vi "UI Allmotion.vi"(8 "error in":errorcluster) -> (0 "error out":errorcluster)   [LabVIEW 2019, in "Allmotion.lvlib"]
uses:
  Allmotion.lvlib
  User Event/Controls/UE Abort Action.ctl
  <vilib>/Utility/miscctls.llb/LVPointTypeDef.ctl
  <vilib>/Utility/error.llb/Error Cluster From Error Code.vi
  <vilib>/Instr/_visa.llb/VISA Configure Serial Port (Instr).vi
  <vilib>/Utility/config.llb/Read Key (String).vi
  <vilib>/ErrorRing/Error Ring.xnode
  Queues/Queues.lvlib
  <vilib>/Utility/config.llb/NI_LVConfig.lvlib
panel:
  in  "Cube":T1(radio)=enum."Cube 1"
  in  "Go Reference":bool
  in  "Joystick Control":T2={"Joystick"=FALSE, "Deadband"={"Axis 1"=2000, "Axis 2"=2000, "Axis 3"=500}, "Multiply"={"Axis 1"=100, "Axis 2"=100, "Axis 3"=25}}
  in  "EMC":bool
  in  "Reset":bool
  in  "Home":bool
  in  "Motion Control":T3
  out "Current Position":i32[](array[numeric])
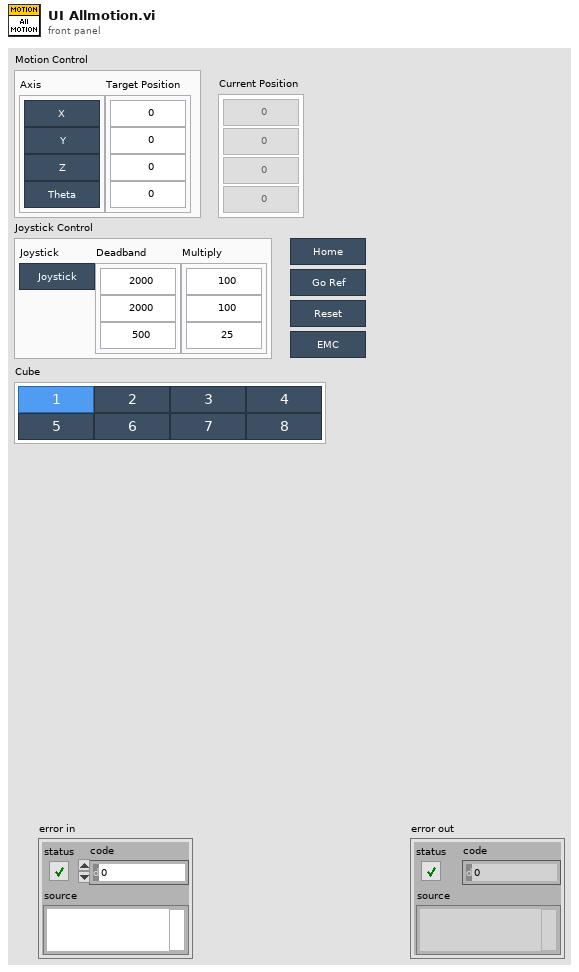
[diagram p1: front panel]
types:
  T1 = enum32{"No Selection", "Cube 1", "Cube 2", "Cube 3", "Cube 4", "Cube 5", "Cube 6", "Cube 7", "Cube 8"}
  T2 = cluster{"Joystick":bool, "Deadband":cluster{"Axis 1":i32, "Axis 2":i32, "Axis 3":i32}, "Multiply":cluster{"Axis 1":i32, "Axis 2":i32, "Axis 3":i32}}
  T3 = cluster{"Axis":cluster{"X":bool, "Y":bool, "Z":bool, "Theta":bool}, "Target Position":cluster{"X":i32, "Y":i32, "Z":i32, "Theta":i32}}
  T4 = cluster{"VISA name":refnum<visa-resource-name>, "Dichroic Position":string[], "Reference":string[]}
  T5 = typedef "UE Abort Action.ctl" = enum16{"Create", "Get", "Destroy"}
  T6 = typedef "LVPointTypeDef.ctl" = cluster{"Horizontal":i16, "Vertical":i16}
  T7 = enum8{"Enabled", "Disabled", "Disabled and Grayed Out"}
  T8 = typedef "NI_LVConfig.lvlib/Config Data RefNum.ctl" = refnum<k1>
  T9 = typedef "Allmotion.lvlib/SEQ Data.ctl" = cluster{"Position":i32[], "Arrived?":bool, "VISA name":refnum<visa-resource-name>, "Initialize Done?":bool, "State":string, "VI Refnum":refnum<vi>, "Dichroic Position":string[]}
  T10 = typedef "Rendezvous RefNum" = refnum<k1>
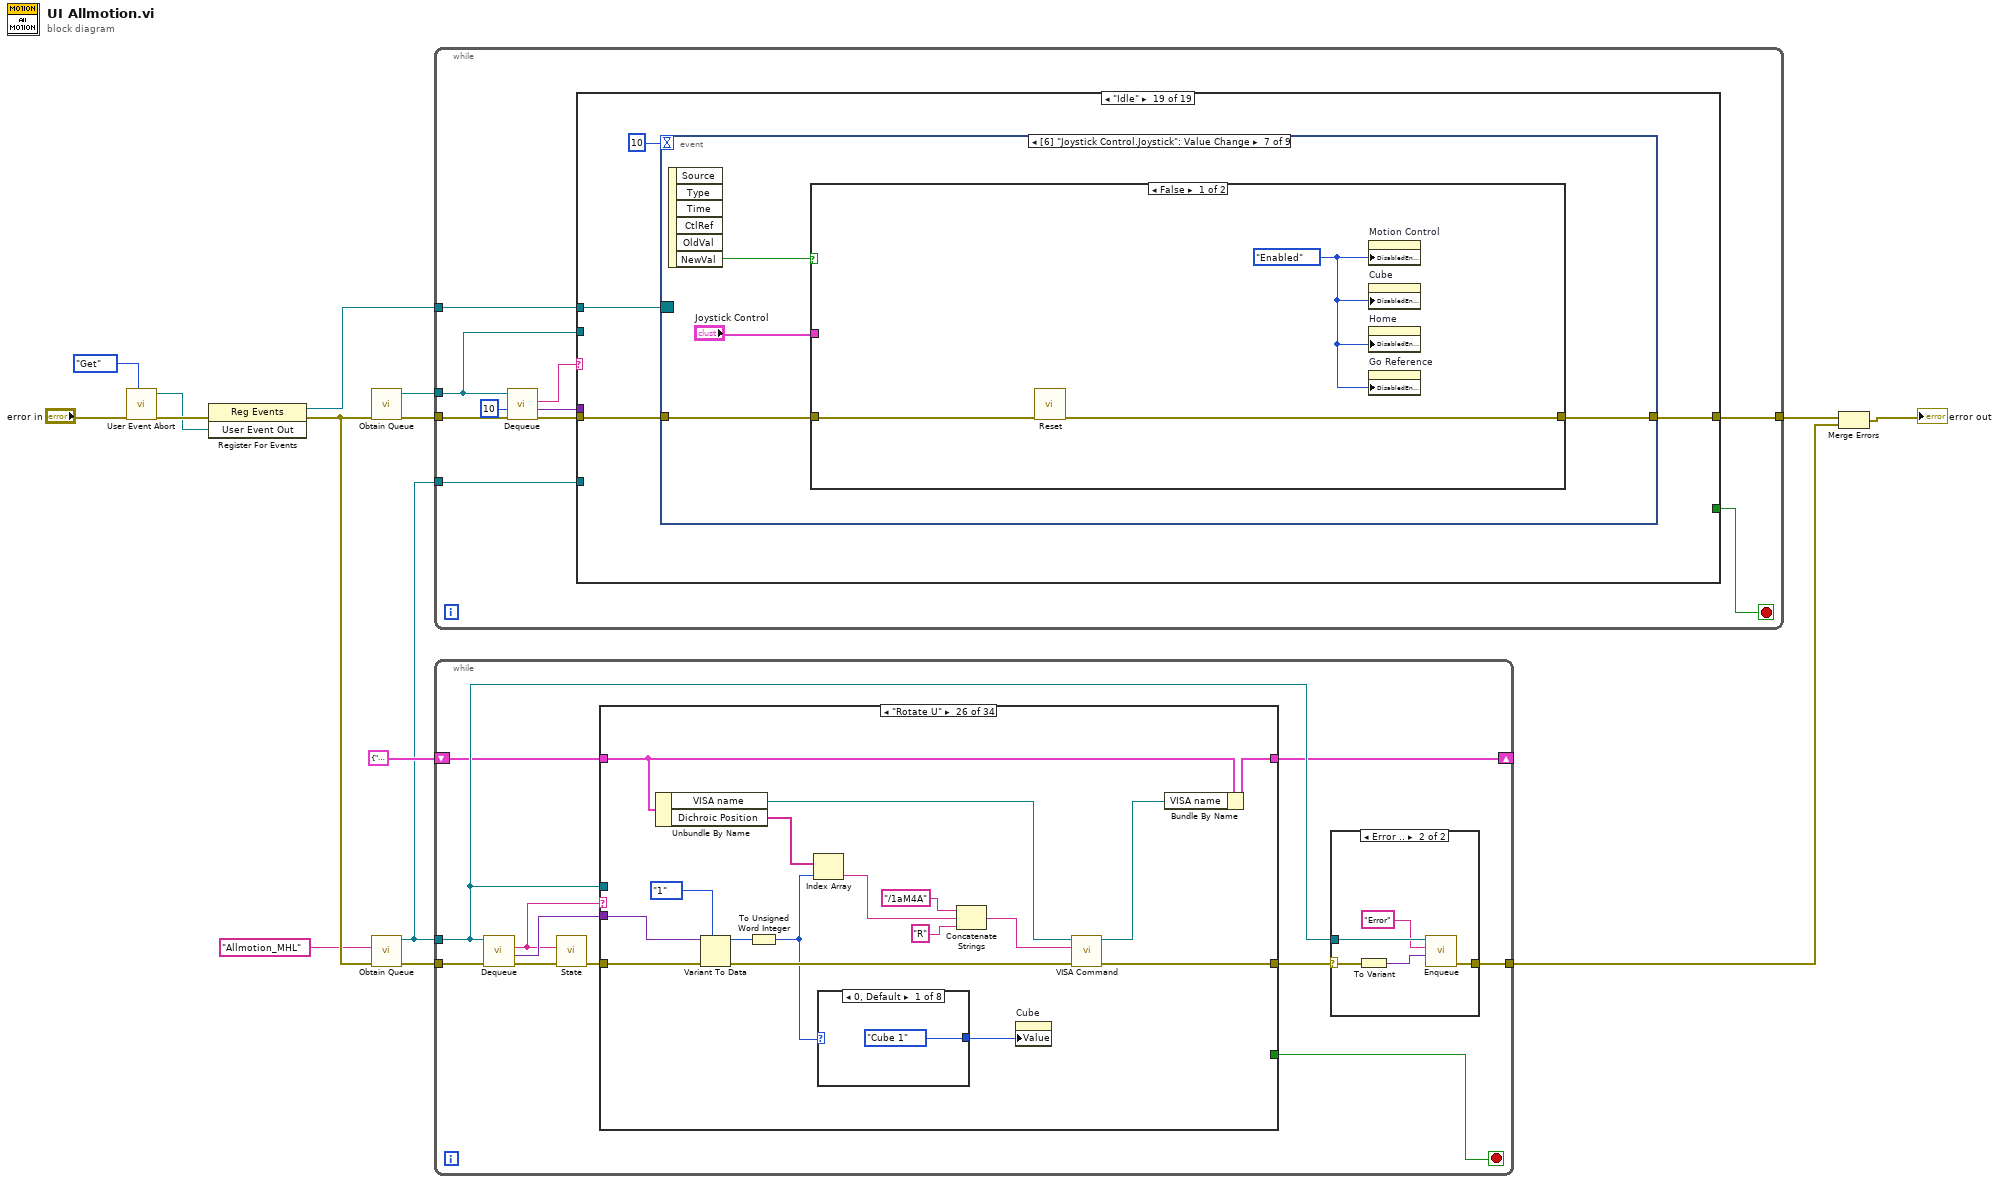
[diagram p0: block diagram]
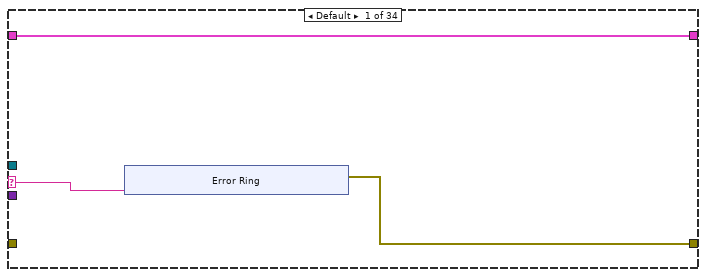
[diagram p3: hidden frame]
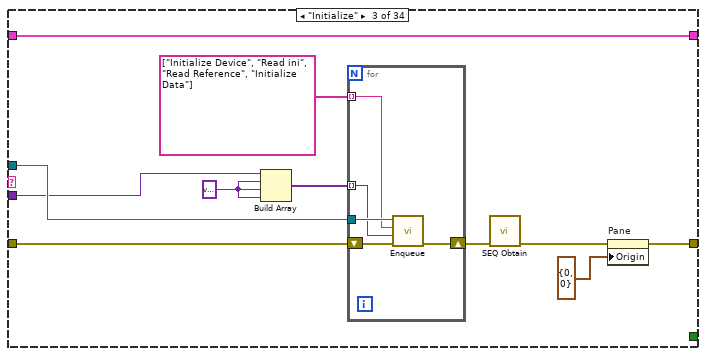
[diagram p5: hidden frame]
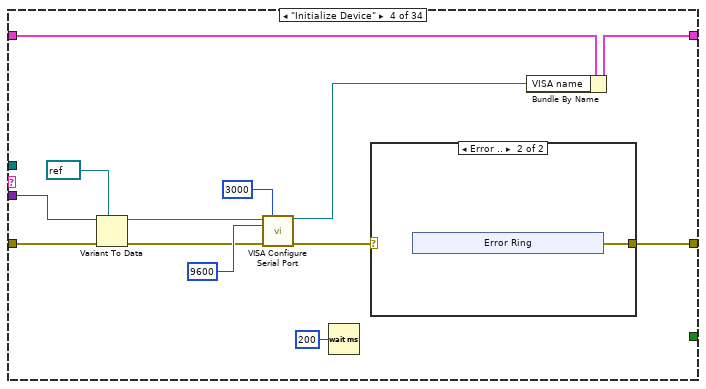
[diagram p6: hidden frame]
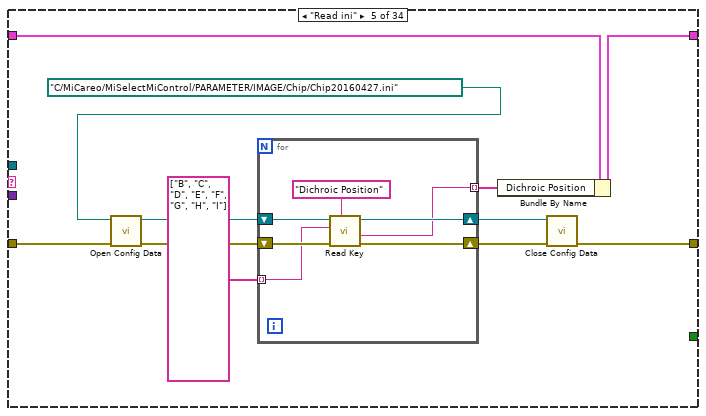
[diagram p8: hidden frame]
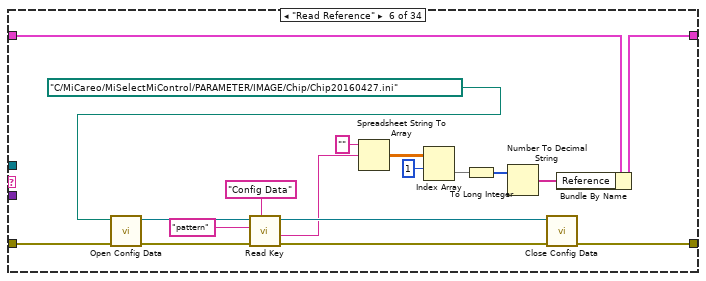
[diagram p9: hidden frame]
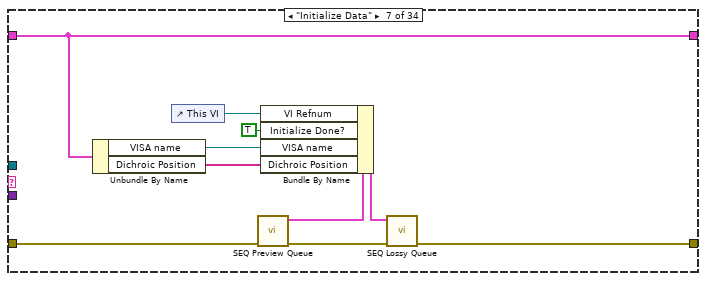
[diagram p10: hidden frame]
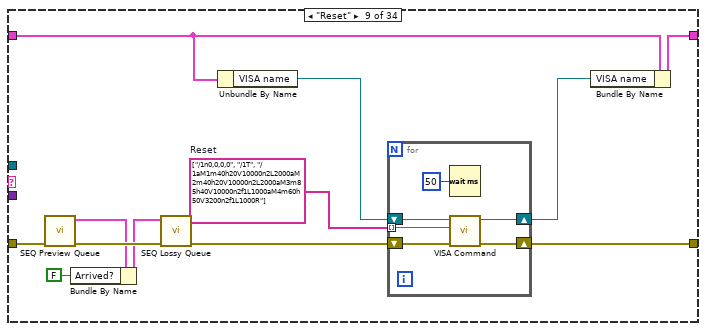
[diagram p12: hidden frame]
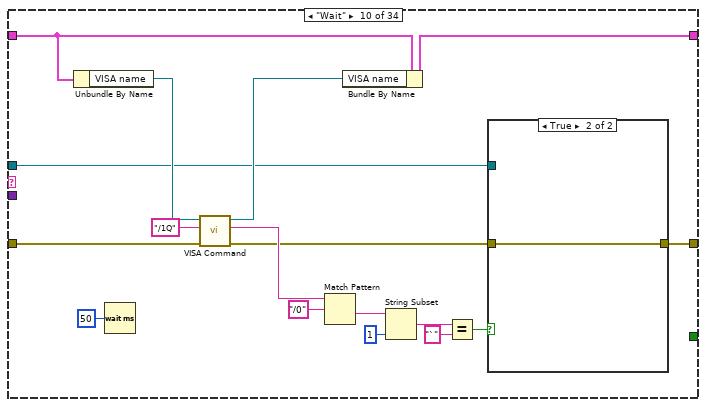
[diagram p13: hidden frame]
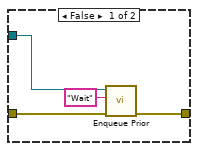
[diagram p14: hidden frame]
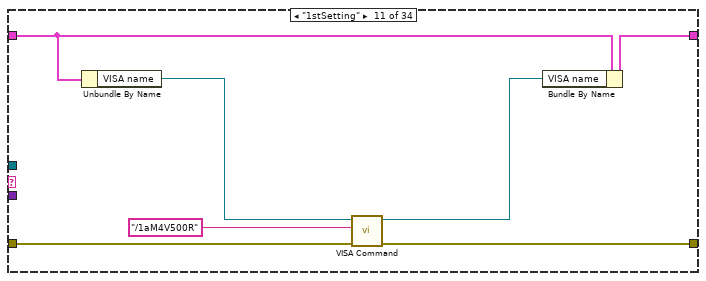
[diagram p15: hidden frame]
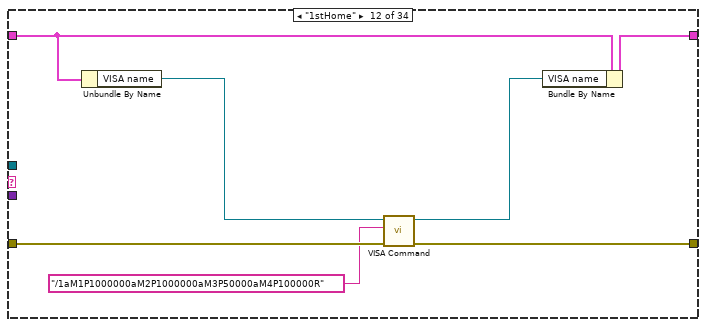
[diagram p16: hidden frame]
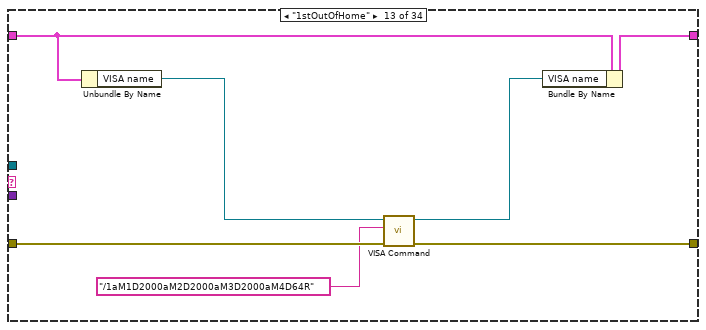
[diagram p17: hidden frame]
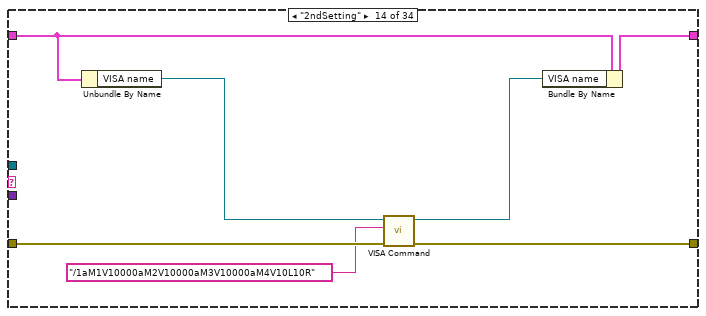
[diagram p18: hidden frame]
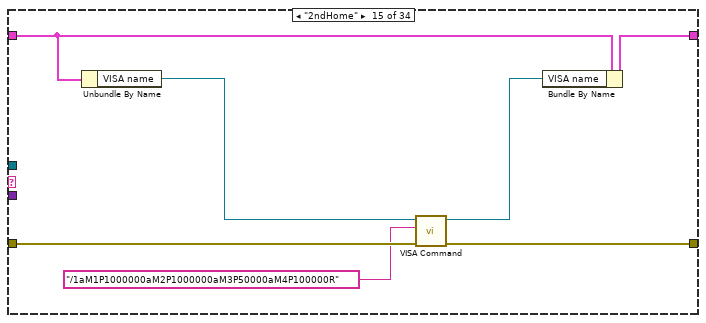
[diagram p19: hidden frame]
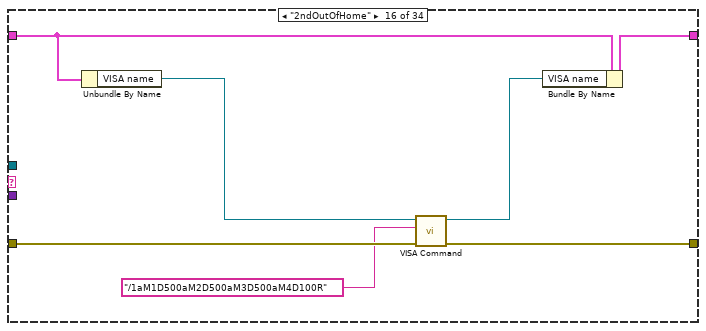
[diagram p20: hidden frame]
diagram:
  n1 = call "User Event Abort.vi"("Action"=UE_Abort_Action."Get", "Error In"="error in") -> ("Error Out"=w13:errorcluster, "User Event Out"=w12:refnum<user-event>)  [unwired: 8 in]
  n2 = register-events(error in=w13, w12) -> (reference out=w11:refnum<event-registration>, error out=w4:errorcluster)  [unwired: 1 in]
  n3 = call "Obtain Queue.vi"("Error In"=w4) -> ("Error Out"=w6:errorcluster, "Queue out"=w5:refnum<queue>)  [unwired: 9 in]
  n4 = call "Obtain Queue.vi"("Error In"=w4, "Queue Name"="Allmotion_MHL") -> ("Error Out"=w3:errorcluster, "queue out"=w2:refnum<queue>)  [unwired: 8 in]
  n5 = while {
    tunnel: w6 -> [w25]
    tunnel: w11 -> [w20]
    tunnel: [w19] -> w10
    tunnel: w2 -> [w17]
    tunnel: w5 -> [w16]
    stop <- w18 stop-if-true
    n6 = call "Dequeue.vi"("Error In"=w25, "timeout in ms (-1)"=10, "Queue in"=w16) -> ("Error Out"=w21:errorcluster, "Data"=w22:variant, "State"=w23:string)  [unwired: 5 in, 1 out]
    n7 = case shown="\"Idle\"" w23 {
      selector: w23 -> [w27 _ _ _ _ _ _ _ _ _ _ _ _ _ _ _ _ _ _]
      tunnel: w22 -> [_ w33 _ w58 _ w92 w113 w134 w155 w166 _ _ w206 _ _ _ _ _ _]
      tunnel: w21 -> [w28 w34 w37 w59 w65 w93 w114 w135 w156 w170 w179 w194 w207 w218 w221 w229 w233 w237 w239]
      tunnel: w20 -> [_ _ _ _ _ _ _ _ _ _ _ _ _ _ _ _ _ _ w241]
      tunnel: [w28 w30 w40 w45 w67 w84 w105 w126 w147 w169 w181 w193 w201 w213 w223 w228 w232 w236 w238] -> w19
      tunnel: [_ _ _ _ _ _ _ _ _ _ _ _ _ _ TRUE _ _ _ _] -> w18
      tunnel: w17 -> [_ w35 w39 w52 w72 w91 w112 w133 w154 w168 w177 w192 w205 w216 w224 w227 w231 w235 _]
      tunnel: w16 -> [_ _ _ _ _ _ _ _ _ _ _ _ _ _ w219 _ _ _ _]
      frame "Typo", Default {
        n8 = Concatenate Strings("Typo: " ("string"), w27) -> (w29:string)
        n9 = One Button Dialog(message=w29) -> ()  [unwired: 1 in, 1 out]
      }
      frame "Initialize" {
        n10 = call "Enqueue.vi"("Error In"=w34, "Data"=w33, "State"="Initialize", "Queue in"=w35) -> ("Error Out"=w31:errorcluster)  [unwired: 6 in, 1 out]
        n11 = property on="Pane" class="Pane"(error in=w31, "Origin"=T6 {"Horizontal"=0, "Vertical"=0}) -> (error out=w30:errorcluster)  [unwired: 1 in, 1 out]
      }
      frame "Home" {
        n12 = for {
          shift-right: [w43] -> w40
          shift-left: w37 -> [w44]
          tunnel: w39 -> [w42]
          tunnel: string[] ["Reset", "Wait", "Wait", "1stSetting", "Wait", "1stHome", "Wait", "1stOutOfHome", "Wait", "2ndSetting", "Wait", "2ndHome", "Wait", "2ndOutOfHome", "Wait", "SetTo0", "Wait", "Wait", "Reset", "Wait", "Position"] -> [w41] mode=indexing
          n13 = call "Enqueue.vi"("Error In"=w44, "State"=w41, "Queue in"=w42) -> ("Error Out"=w43:errorcluster)  [unwired: 7 in, 1 out]
        }
      }
      frame "Move" {
        w47 = variant ("variant")
        n14 = Variant To Data(error in=w59, type=i32[] [] ("4position"), Variant=w58) -> (data=w55:i32[], error out=w56:errorcluster)
        n15 = call "Convert Move Command.vi"("error in"=w56, "Position in"=w55) -> ("error out"=w53:errorcluster, "Command out"=w54:string)  [unwired: 8 in]
        n16 = To Variant(anything=w54) -> (Variant=w50:variant)
        n17 = To Variant(anything=u32 50 ("milliseconds to wait")) -> (Variant=w49:variant)
        n18 = Build Array(w47, w50, w47, w49, w47) -> (w46:variant[])
        n19 = for {
          tunnel: w52 -> [w63]
          tunnel: string[] ["Reset", "Move", "Wait", "Delay", "Position"] -> [w62] mode=indexing
          tunnel: w46 -> [w61] mode=indexing
          shift-right: [w60] -> w45
          shift-left: w53 -> [w64]
          n20 = call "Enqueue.vi"("Error In"=w64, "Data"=w61, "State"=w62, "Queue in"=w63) -> ("Error Out"=w60:errorcluster)  [unwired: 6 in, 1 out]
        }
      }
      frame "Go Reference" {
        w66 = variant ("variant")
        n21 = To Variant(anything=u32 50 ("milliseconds to wait")) -> (Variant=w70:variant)
        n22 = Build Array(w66, w66, w66, w70, w66) -> (w68:variant[])
        n23 = for {
          tunnel: w72 -> [w76]
          tunnel: string[] ["Reset", "Go Reference", "Wait", "Delay", "Position"] -> [w75] mode=indexing
          tunnel: w68 -> [w74] mode=indexing
          shift-right: [w73] -> w67
          shift-left: w65 -> [w77]
          n24 = call "Enqueue.vi"("Error In"=w77, "Data"=w74, "State"=w75, "Queue in"=w76) -> ("Error Out"=w73:errorcluster)  [unwired: 6 in, 1 out]
        }
      }
      frame "Move Axis 1" {
        w86 = variant ("variant")
        n25 = Variant To Data(error in=w93, type="", Variant=w92) -> (data=w79:string, error out=w83:errorcluster)
        n26 = Concatenate Strings("/1aM1A", w79, "R" ("string")) -> (w78:string)
        n27 = To Variant(anything=w78) -> (Variant=w89:variant)
        n28 = To Variant(anything=u32 50 ("milliseconds to wait")) -> (Variant=w88:variant)
        n29 = Build Array(w86, w89, w86, w88, w86) -> (w85:variant[])
        n30 = for {
          tunnel: w91 -> [w97]
          tunnel: string[] ["Reset", "Move", "Wait", "Delay", "Position"] -> [w96] mode=indexing
          tunnel: w85 -> [w95] mode=indexing
          shift-right: [w94] -> w84
          shift-left: w83 -> [w98]
          n31 = call "Enqueue.vi"("Error In"=w98, "Data"=w95, "State"=w96, "Queue in"=w97) -> ("Error Out"=w94:errorcluster)  [unwired: 6 in, 1 out]
        }
      }
      frame "Move Axis 2" {
        w107 = variant ("variant")
        n32 = Variant To Data(error in=w114, type="", Variant=w113) -> (data=w100:string, error out=w104:errorcluster)
        n33 = Concatenate Strings("/1aM2A", w100, "R" ("string")) -> (w99:string)
        n34 = To Variant(anything=w99) -> (Variant=w110:variant)
        n35 = To Variant(anything=u32 50 ("milliseconds to wait")) -> (Variant=w109:variant)
        n36 = Build Array(w107, w110, w107, w109, w107) -> (w106:variant[])
        n37 = for {
          tunnel: w112 -> [w118]
          tunnel: string[] ["Reset", "Move", "Wait", "Delay", "Position"] -> [w117] mode=indexing
          tunnel: w106 -> [w116] mode=indexing
          shift-right: [w115] -> w105
          shift-left: w104 -> [w119]
          n38 = call "Enqueue.vi"("Error In"=w119, "Data"=w116, "State"=w117, "Queue in"=w118) -> ("Error Out"=w115:errorcluster)  [unwired: 6 in, 1 out]
        }
      }
      frame "Move Axis 3" {
        w128 = variant ("variant")
        n39 = Variant To Data(error in=w135, type="", Variant=w134) -> (data=w121:string, error out=w125:errorcluster)
        n40 = Concatenate Strings("/1aM3A", w121, "R" ("string")) -> (w120:string)
        n41 = To Variant(anything=w120) -> (Variant=w131:variant)
        n42 = To Variant(anything=u32 50 ("milliseconds to wait")) -> (Variant=w130:variant)
        n43 = Build Array(w128, w131, w128, w130, w128) -> (w127:variant[])
        n44 = for {
          tunnel: w133 -> [w139]
          tunnel: string[] ["Reset", "Move", "Wait", "Delay", "Position"] -> [w138] mode=indexing
          tunnel: w127 -> [w137] mode=indexing
          shift-right: [w136] -> w126
          shift-left: w125 -> [w140]
          n45 = call "Enqueue.vi"("Error In"=w140, "Data"=w137, "State"=w138, "Queue in"=w139) -> ("Error Out"=w136:errorcluster)  [unwired: 6 in, 1 out]
        }
      }
      frame "Move Axis 4" {
        w149 = variant ("variant")
        n46 = Variant To Data(error in=w156, type="", Variant=w155) -> (data=w142:string, error out=w146:errorcluster)
        n47 = Concatenate Strings("/1aM4A", w142, "R" ("string")) -> (w141:string)
        n48 = To Variant(anything=w141) -> (Variant=w152:variant)
        n49 = To Variant(anything=u32 50 ("milliseconds to wait")) -> (Variant=w151:variant)
        n50 = Build Array(w149, w152, w149, w151, w149) -> (w148:variant[])
        n51 = for {
          tunnel: w154 -> [w160]
          tunnel: string[] ["Reset", "Move", "Wait", "Delay", "Position"] -> [w159] mode=indexing
          tunnel: w148 -> [w158] mode=indexing
          shift-right: [w157] -> w147
          shift-left: w146 -> [w161]
          n52 = call "Enqueue.vi"("Error In"=w161, "Data"=w158, "State"=w159, "Queue in"=w160) -> ("Error Out"=w157:errorcluster)  [unwired: 6 in, 1 out]
        }
      }
      frame "Rotate U" {
        w165 = variant
        n53 = To Variant(anything=u32 50 ("milliseconds to wait")) -> (Variant=w162:variant)
        n54 = Build Array(w165, w166, w165, w162, w165) -> (w164:variant[])
        n55 = for {
          tunnel: w168 -> [w173]
          shift-right: [w174] -> w169
          shift-left: w170 -> [w175]
          tunnel: string[] ["Reset", "Rotate U", "Wait", "Delay", "Position"] -> [w172] mode=indexing
          tunnel: w164 -> [w171] mode=indexing
          n56 = call "Enqueue.vi"("Error In"=w175, "Data"=w171, "State"=w172, "Queue in"=w173) -> ("Error Out"=w174:errorcluster)  [unwired: 6 in, 1 out]
        }
      }
      frame "Reset" {
        w180 = variant ("variant")
        n57 = Flush Queue(queue=w177, error in (no error)=w179) -> (queue out=w176:refnum<queue>, error out=w178:errorcluster)  [unwired: 1 out]
        n58 = To Variant(anything=u32 50 ("milliseconds to wait")) -> (Variant=w184:variant)
        n59 = Build Array(w180, w180, w184, w180) -> (w182:variant[])
        n60 = for {
          tunnel: string[] ["Reset", "Wait", "Delay", "Position"] -> [w189] mode=indexing
          tunnel: w182 -> [w188] mode=indexing
          shift-right: [w187] -> w181
          shift-left: w178 -> [w190]
          tunnel: w176 -> [w186]
          n61 = call "Enqueue.vi"("Error In"=w190, "Data"=w188, "State"=w189, "Queue in"=w186) -> ("Error Out"=w187:errorcluster)  [unwired: 6 in, 1 out]
        }
      }
      frame "Position" {
        n62 = call "Enqueue.vi"("Error In"=w194, "State"="Position", "Queue in"=w192) -> ("Error Out"=w193:errorcluster)  [unwired: 7 in, 1 out]
      }
      frame "Joystick" {
        w195 = variant ("variant")
        n63 = Variant To Data(error in=w207, type="", Variant=w206) -> (data=w198:string, error out=w199:errorcluster)
        n64 = To Variant(anything=w198) -> (Variant=w197:variant)
        n65 = To Variant(anything=u32 50 ("milliseconds to wait")) -> (Variant=w196:variant)
        n66 = Build Array(w195, w195, w197, w196, w195) -> (w202:variant[])
        n67 = for {
          tunnel: w205 -> [w211]
          tunnel: string[] ["Reset", "Wait", "Joystick", "Delay", "Position Continue"] -> [w210] mode=indexing
          tunnel: w202 -> [w209] mode=indexing
          shift-right: [w208] -> w201
          shift-left: w199 -> [w212]
          n68 = call "Enqueue.vi"("Error In"=w212, "Data"=w209, "State"=w210, "Queue in"=w211) -> ("Error Out"=w208:errorcluster)  [unwired: 6 in, 1 out]
        }
      }
      frame "Emergency Stop" {
        n69 = Flush Queue(queue=w216, error in (no error)=w218) -> (queue out=w215:refnum<queue>, error out=w217:errorcluster)  [unwired: 1 out]
        n70 = call "Enqueue.vi"("Error In"=w217, "State"="Emergency Stop", "Queue in"=w215) -> ("Error Out"=w213:errorcluster)  [unwired: 7 in, 1 out]
      }
      frame "Close" {
        n71 = Release Queue(queue=w219, error in (no error)=w221) -> (error out=w220:errorcluster)  [unwired: 1 in, 2 out]
        n72 = call "Enqueue.vi"("Error In"=w220, "State"="Close", "Queue in"=w224) -> ("Error Out"=w223:errorcluster)  [unwired: 7 in, 1 out]
      }
      frame "Rendezvous Acquire" {
        n73 = call "Enqueue.vi"("Error In"=w229, "State"="Rendezvous Acquire", "Queue in"=w227) -> ("Error Out"=w228:errorcluster)  [unwired: 7 in, 1 out]
      }
      frame "Rendezvous Focus" {
        n74 = call "Enqueue.vi"("Error In"=w233, "State"="Rendezvous Focus", "Queue in"=w231) -> ("Error Out"=w232:errorcluster)  [unwired: 7 in, 1 out]
      }
      frame "Rendezvous Align" {
        n75 = call "Enqueue.vi"("Error In"=w237, "State"="Rendezvous Align", "Queue in"=w235) -> ("Error Out"=w236:errorcluster)  [unwired: 7 in, 1 out]
      }
      frame "Idle" {
        n76 = event shown="[6] \"Joystick Control.Joystick\": Value Change" {
          selector: w241 -> [_ _ _ _ _ _ _ _ w330]
          dyn-events: _ -> [_ _ _ _ _ _ _ _ _]
          timeout: 10 -> [_ _ _ _ _ _ _ _ _]
          tunnel: w239 -> [w242 w244 w270 w272 w274 w276 w280 w304 w333]
          tunnel: [w242 w243 w269 w271 w273 w275 w277 w303 w331] -> w238
          event Timeout {
            n77 = event-data() -> ()  [unwired: 1 in, 3 out]
          }
          event "Motion Control.Axis.X", "Motion Control.Axis.Y", "Motion Control.Axis.Z", "Motion Control.Axis.Theta": Value Change {
            n78 = event-data() -> ("CtlRef"=w247:refnum<vi>)  [unwired: 1 in, 5 out]
            n79 = property class="Bool"(reference=w247) -> ("Label.Text"=w246:string)  [unwired: 1 in, 2 out]
            n80 = case shown="\"Theta\"" w246 {
              tunnel: "Motion Control" -> [_ w253 w258 w263 w268]
              tunnel: w244 -> [w248 w250 w256 w261 w266]
              tunnel: [w248 w249 w255 w260 w265] -> w243
              frame Default {
              }
              frame "X" {
                n81 = Unbundle By Name(w253) -> ("Target Position.X"=w252:i32)
                n82 = Number To Decimal String(number=w252) -> (decimal integer string=w251:string)  [unwired: 1 in]
                n83 = call "Move Axis 1.vi"("Error In"=w250, "Position"=w251) -> ("Error Out"=w249:errorcluster)  [unwired: 9 in]
              }
              frame "Y" {
                n84 = Unbundle By Name(w258) -> ("Target Position.Y"=w257:i32)
                n85 = Number To Decimal String(number=w257) -> (decimal integer string=w254:string)  [unwired: 1 in]
                n86 = call "Move Axis 2.vi"("Error In"=w256, "Position"=w254) -> ("Error Out"=w255:errorcluster)  [unwired: 9 in]
              }
              frame "Z" {
                n87 = Unbundle By Name(w263) -> ("Target Position.Z"=w262:i32)
                n88 = Number To Decimal String(number=w262) -> (decimal integer string=w259:string)  [unwired: 1 in]
                n89 = call "Move Axis 3.vi"("Error In"=w261, "Position"=w259) -> ("Error Out"=w260:errorcluster)  [unwired: 9 in]
              }
              frame "Theta" {
                n90 = Unbundle By Name(w268) -> ("Target Position.Theta"=w267:i32)
                n91 = Number To Decimal String(number=w267) -> (decimal integer string=w264:string)  [unwired: 1 in]
                n92 = call "Move Axis 4.vi"("Error In"=w266, "Position"=w264) -> ("Error Out"=w265:errorcluster)  [unwired: 9 in]
              }
            }
          }
          event "Home": Value Change {
            n93 = event-data() -> ()  [unwired: 1 in, 6 out]
            n94 = call "Home.vi"("Error In"=w270) -> ("Error Out"=w269:errorcluster)  [unwired: 10 in]
          }
          event "Go Reference": Value Change {
            n95 = event-data() -> ()  [unwired: 1 in, 6 out]
            n96 = call "Go Reference.vi"("Error In"=w272) -> ("Error Out"=w271:errorcluster)  [unwired: 10 in]
          }
          event "Reset": Value Change {
            n97 = event-data() -> ()  [unwired: 1 in, 6 out]
            n98 = call "Reset.vi"("Error In"=w274) -> ("Error Out"=w273:errorcluster)  [unwired: 10 in]
          }
          event "EMC": Value Change {
            n99 = event-data() -> ()  [unwired: 1 in, 6 out]
            n100 = call "Emergency Stop.vi"("Error In"=w276) -> ("Error Out"=w275:errorcluster)  [unwired: 10 in]
          }
          event "Joystick Control.Joystick": Value Change {
            n101 = event-data() -> ("NewVal"=w279:bool)  [unwired: 1 in, 5 out]
            n102 = case shown="False" w279 {
              tunnel: w280 -> [w283 w287]
              tunnel: "Joystick Control" -> [_ w301]
              tunnel: [w282 w286] -> w277
              frame False {
                w281 = T7."Enabled" ("Disabled")
                n103 = call "Reset.vi"("Error In"=w283) -> ("Error Out"=w282:errorcluster)  [unwired: 10 in]
                n104 = property on="Motion Control" class="Clust"("DisabledEnum"=w281) -> ()  [unwired: 2 in, 2 out]
                n105 = property on="Cube" class="RadioBtnsControl (strict)"("DisabledEnum"=w281) -> ()  [unwired: 2 in, 2 out]
                n106 = property on="Home" class="Bool"("DisabledEnum"=w281) -> ()  [unwired: 2 in, 2 out]
                n107 = property on="Go Reference" class="Bool"("DisabledEnum"=w281) -> ()  [unwired: 2 in, 2 out]
              }
              frame True {
                w284 = T7."Disabled and Grayed Out" ("Disabled")
                n108 = Unbundle By Name(w301) -> ("Deadband.Axis 1"=w299:i32, "Deadband.Axis 2"=w298:i32, "Deadband.Axis 3"=w297:i32, "Multiply.Axis 1"=w296:i32, "Multiply.Axis 2"=w295:i32, "Multiply.Axis 3"=w294:i32)
                n109 = Number To Decimal String(number=w299) -> (decimal integer string=w293:string)  [unwired: 1 in]
                n110 = Number To Decimal String(number=w298) -> (decimal integer string=w292:string)  [unwired: 1 in]
                n111 = Number To Decimal String(number=w297) -> (decimal integer string=w291:string)  [unwired: 1 in]
                n112 = Number To Decimal String(number=w296) -> (decimal integer string=w290:string)  [unwired: 1 in]
                n113 = Number To Decimal String(number=w295) -> (decimal integer string=w289:string)  [unwired: 1 in]
                n114 = Number To Decimal String(number=w294) -> (decimal integer string=w288:string)  [unwired: 1 in]
                n115 = Format Into String(format string="/1n65538,65538,65538,ad%s,%s,%s,am%s,%s,%s,z0,0,0,P0,0,0,R", w293, w292, w291, w290, w289, w288) -> (resulting string=w285:string)  [unwired: 2 in, 1 out]
                n116 = call "Joystick.vi"("Error In"=w287, "Command"=w285) -> ("Error Out"=w286:errorcluster)  [unwired: 9 in]
                n117 = property on="Motion Control" class="Clust"("DisabledEnum"=w284) -> ()  [unwired: 2 in, 2 out]
                n118 = property on="Cube" class="RadioBtnsControl (strict)"("DisabledEnum"=w284) -> ()  [unwired: 2 in, 2 out]
                n119 = property on="Home" class="Bool"("DisabledEnum"=w284) -> ()  [unwired: 2 in, 2 out]
                n120 = property on="Go Reference" class="Bool"("DisabledEnum"=w284) -> ()  [unwired: 2 in, 2 out]
              }
            }
          }
          event "Cube": Value Change {
            n121 = event-data() -> ("NewVal"=w302:T1)  [unwired: 1 in]
            n122 = case shown="\"No Selection\", Default" w302 {
              tunnel: w304 -> [w305 w308 w311 w314 w317 w320 w323 w326 w329]
              tunnel: [w305 w307 w310 w313 w316 w319 w322 w325 w328] -> w303
              frame "No Selection", Default {
              }
              frame "Cube 1" {
                n123 = call "Rotate U.vi"("Error In"=w308, "Cube"=enum16{"1", "2", "3", "4", "5", "6", "7", "8"}."1") -> ("Error Out"=w307:errorcluster)  [unwired: 9 in]
              }
              frame "Cube 2" {
                n124 = call "Rotate U.vi"("Error In"=w311, "Cube"=enum16{"1", "2", "3", "4", "5", "6", "7", "8"}."2") -> ("Error Out"=w310:errorcluster)  [unwired: 9 in]
              }
              frame "Cube 3" {
                n125 = call "Rotate U.vi"("Error In"=w314, "Cube"=enum16{"1", "2", "3", "4", "5", "6", "7", "8"}."3") -> ("Error Out"=w313:errorcluster)  [unwired: 9 in]
              }
              frame "Cube 4" {
                n126 = call "Rotate U.vi"("Error In"=w317, "Cube"=enum16{"1", "2", "3", "4", "5", "6", "7", "8"}."4") -> ("Error Out"=w316:errorcluster)  [unwired: 9 in]
              }
              frame "Cube 5" {
                n127 = call "Rotate U.vi"("Error In"=w320, "Cube"=enum16{"1", "2", "3", "4", "5", "6", "7", "8"}."5") -> ("Error Out"=w319:errorcluster)  [unwired: 9 in]
              }
              frame "Cube 6" {
                n128 = call "Rotate U.vi"("Error In"=w323, "Cube"=enum16{"1", "2", "3", "4", "5", "6", "7", "8"}."6") -> ("Error Out"=w322:errorcluster)  [unwired: 9 in]
              }
              frame "Cube 7" {
                n129 = call "Rotate U.vi"("Error In"=w326, "Cube"=enum16{"1", "2", "3", "4", "5", "6", "7", "8"}."7") -> ("Error Out"=w325:errorcluster)  [unwired: 9 in]
              }
              frame "Cube 8" {
                n130 = call "Rotate U.vi"("Error In"=w329, "Cube"=enum16{"1", "2", "3", "4", "5", "6", "7", "8"}."8") -> ("Error Out"=w328:errorcluster)  [unwired: 9 in]
              }
            }
          }
          event User Event {
            n131 = event-data() -> ()  [unwired: 1 in, 4 out]
            n132 = call "Close.vi"("Error In"=w333) -> ("Error Out"=w332:errorcluster)  [unwired: 10 in]
            n133 = Unregister For Events(event registration refnum=w330, error in=w332) -> (error out=w331:errorcluster)
          }
        }
      }
    }
  }
  n134 = while {
    tunnel: w3 -> [w344]
    tunnel: w2 -> [w339]
    tunnel: [w340] -> w8
    shift-right: [w337] -> _
    shift-left: T4 {"VISA name"="", "Dichroic Position"=[], "Reference"=[]} -> [w338]
    stop <- w342 stop-if-true
    n135 = call "Dequeue.vi"("Error In"=w344, "Queue in"=w339) -> ("Error Out"=w336:errorcluster, "Data"=w343:variant, "State"=w334:string)  [unwired: 6 in, 1 out]
    n136 = call "State.vi"("error in"=w336, "State"=w334) -> ("error out"=w335:errorcluster)  [unwired: 9 in]
    n137 = case shown="\"Rotate U\"" w334 {
      selector: w334 -> [w353 _ _ _ _ _ _ _ _ _ _ _ _ _ _ _ _ _ _ _ _ _ _ _ _ _ _ _ _ _ _ _ _ _]
      tunnel: w343 -> [_ _ w365 w381 _ _ _ _ _ _ _ _ _ _ _ _ _ _ w553 w563 w574 _ _ _ _ w645 _ _ _ w697 _ _ _ _]
      tunnel: w335 -> [_ w362 w373 w383 w403 w429 w437 w446 w448 w481 w493 w500 w507 w514 w521 w528 w535 w550 w555 w565 w575 w579 w593 w610 w627 w647 w665 w686 w693 w698 w701 w706 w714 w720]
      tunnel: w339 -> [_ _ w372 _ _ _ _ _ _ w465 _ _ _ _ _ _ _ _ _ _ _ _ _ _ _ _ w663 _ _ _ _ w704 _ w719]
      tunnel: [w352 w362 w367 w384 w402 w428 w439 w446 w458 w466 w492 w499 w506 w513 w520 w527 w534 w543 w560 w570 w573 w584 w585 w602 w619 w652 w672 w691 w693 errorcluster {"status"=FALSE, "code"=0, "source"=""} ("error constant") w701 w705 w713 w715] -> w341
      tunnel: [_ _ _ _ _ _ _ _ _ _ _ _ _ _ _ _ _ _ _ _ _ _ _ _ _ _ _ _ _ _ _ _ _ TRUE] -> w342
      tunnel: w338 -> [w351 w361 w370 w391 w409 w434 w441 w445 w457 w480 w491 w498 w505 w512 w519 w526 w533 w549 w559 w569 w576 w583 w594 w611 w628 w651 w678 w690 w692 w699 w700 w702 w712 w717]
      tunnel: [w351 w361 w370 w387 w401 w427 w441 w445 w456 w479 w490 w497 w504 w511 w518 w525 w532 w548 w558 w568 w576 w582 w594 w611 w628 w650 w677 w689 w692 w699 w700 w702 w712 w717] -> w337
      frame Default {
        n138 = xnode "Error Ring"("parameter 0"=w353) -> ("error out"=w352:errorcluster)
      }
      frame "------Initialize------" {
      }
      frame "Initialize" {
        w363 = variant
        n139 = Build Array(w365, w363, w363, w363) -> (w364:variant[])
        n140 = for {
          tunnel: w372 -> [w376]
          shift-right: [w377] -> w369
          shift-left: w373 -> [w378]
          tunnel: string[] ["Initialize Device", "Read ini", "Read Reference", "Initialize Data"] -> [w375] mode=indexing
          tunnel: w364 -> [w374] mode=indexing
          n141 = call "Enqueue.vi"("Error In"=w378, "Data"=w374, "State"=w375, "Queue in"=w376) -> ("Error Out"=w377:errorcluster)  [unwired: 6 in, 1 out]
        }
        n142 = call "SEQ Obtain.vi"("error in"=w369) -> ("error out"=w368:errorcluster)  [unwired: 9 in, 1 out]
        n143 = property on="Pane" class="Pane"(error in=w368, "Origin"=T6 {"Horizontal"=0, "Vertical"=0}) -> (error out=w367:errorcluster)  [unwired: 1 in, 1 out]
      }
      frame "Initialize Device" {
        n144 = Variant To Data(error in=w383, type=refnum<visa-resource-name> refnum ("VISA resource name out"), Variant=w381) -> (data=w379:refnum<visa-resource-name>, error out=w380:errorcluster)
        n145 = call-poly "VISA Configure Serial Port"("VISA resource name"=w379, "timeout (10sec)"=u32 3000, "baud rate (9600)"=u32 9600, "error in (no error)"=w380) -> ("VISA resource name out"=w386:refnum<visa-resource-name>, "error out"=w385:errorcluster)  [unwired: 10 in]
        n146 = Wait (ms)(milliseconds to wait=u32 200) -> ()  [unwired: 1 out]
        n147 = case shown="Error .." w385 {
          selector: w385 -> [w392 _]
          tunnel: [w392 w393] -> w384
          frame No Error {
          }
          frame Error {
            n148 = xnode "Error Ring"() -> ("error out"=w393:errorcluster)
          }
        }
        n149 = Bundle By Name(cluster=w391, "VISA name"=w386) -> (w387:T4)
      }
      frame "Read ini" {
        n150 = call <vilib>:"Open Config Data.vi"("error in (no error)"=w403, "configuration file path"=path "C:/MiCareo/MiSelectMiControl/PARAMETER/IMAGE/Chip/Chip20160427.ini") -> ("error out"=w408:errorcluster, "refnum"=w406:T8)  [unwired: 7 in, 1 out]
        n151 = for {
          shift-right: [w415] -> w407
          shift-left: w408 -> [w416]
          shift-right: [w413] -> w405
          shift-left: w406 -> [w414]
          tunnel: string[] ["B", "C", "D", "E", "F", "G", "H", "I"] ("Array") -> [w411] mode=indexing
          tunnel: [w410] -> w400 mode=indexing
          n152 = call-poly <vilib>:"Read Key.vi"("section"="Dichroic Position", "error in (no error)"=w416, "key"=w411, "refnum"=w414) -> ("error out"=w415:errorcluster, "value"=w410:string, "refnum out"=w413:T8)  [unwired: 4 in, 1 out]
        }
        n153 = Bundle By Name(cluster=w409, "Dichroic Position"=w400) -> (w401:T4)
        n154 = call <vilib>:"Close Config Data.vi"("error in (no error)"=w407, "refnum"=w405) -> ("error out"=w402:errorcluster)  [unwired: 8 in, 1 out]
      }
      frame "Read Reference" {
        n155 = call <vilib>:"Open Config Data.vi"("error in (no error)"=w429, "configuration file path"=path "C:/MiCareo/MiSelectMiControl/PARAMETER/IMAGE/Chip/Chip20160427.ini") -> ("error out"=w433:errorcluster, "refnum"=w431:T8)  [unwired: 7 in, 1 out]
        n156 = call-poly <vilib>:"Read Key.vi"("section"="Config Data", "error in (no error)"=w433, "key"="pattern", "refnum"=w431) -> ("error out"=w432:errorcluster, "value"=w421:string, "refnum out"=w430:T8)  [unwired: 4 in, 1 out]
        n157 = Spreadsheet String To Array(format string="", spreadsheet string=w421) -> (array=w420:dbl[][])  [unwired: 2 in]
        n158 = Index Array(array=w420, index (row)=1) -> (element=w419:dbl[])  [unwired: 1 in]
        n159 = To Long Integer(number=w419) -> (32bit integer=w418:i32[])
        n160 = Number To Decimal String(number=w418) -> (decimal integer string=w417:string[])  [unwired: 1 in]
        n161 = call <vilib>:"Close Config Data.vi"("error in (no error)"=w432, "refnum"=w430) -> ("error out"=w428:errorcluster)  [unwired: 8 in, 1 out]
        n162 = Bundle By Name(cluster=w434, "Reference"=w417) -> (w427:T4)
      }
      frame "Initialize Data" {
        n163 = Unbundle By Name(w441) -> ("VISA name"=w440:refnum<visa-resource-name>, "Dichroic Position"=w435:string[])
        n164 = control-ref of="This VI"() -> (w436:refnum<vi>)
        n165 = call "SEQ Preview Queue.vi"("error in"=w437) -> ("error out"=w444:errorcluster, "SEQ Data"=w443:T9)  [unwired: 9 in]
        n166 = Bundle By Name(cluster=w443, "VI Refnum"=w436, "Initialize Done?"=TRUE, "VISA name"=w440, "Dichroic Position"=w435) -> (w442:T9)
        n167 = call "SEQ Lossy Queue.vi"("error in"=w444, "SEQ Data"=w442) -> ("error out"=w439:errorcluster)  [unwired: 9 in]
      }
      frame "------Functions------" {
      }
      frame "Reset" {
        w453 = string[] ["/1n0,0,0,0", "/1T", "/1aM1m40h20V10000n2L2000aM2m40h20V10000n2L2000aM3m85h40V10000n2f1L1000aM4m60h50V3200n2f1L1000R"]  # Reset
        n168 = call "SEQ Preview Queue.vi"("error in"=w448) -> ("error out"=w452:errorcluster, "SEQ Data"=w451:T9)  [unwired: 9 in]
        n169 = Bundle By Name(cluster=w451, "Arrived?"=FALSE) -> (w450:T9)
        n170 = call "SEQ Lossy Queue.vi"("error in"=w452, "SEQ Data"=w450) -> ("error out"=w447:errorcluster)  [unwired: 9 in]
        n171 = Unbundle By Name(w457) -> ("VISA name"=w455:refnum<visa-resource-name>)
        n172 = for {
          shift-right: [w463] -> w458
          shift-left: w447 -> [w464]
          shift-right: [w461] -> w454
          shift-left: w455 -> [w462]
          tunnel: w453 -> [w460] mode=indexing
          n173 = Wait (ms)(milliseconds to wait=u32 50) -> ()  [unwired: 1 out]
          n174 = call "VISA Command.vi"("error in"=w464, "Command"=w460, "VISA name in"=w462) -> ("error out"=w463:errorcluster, "VISA name out"=w461:refnum<visa-resource-name>)  [unwired: 6 in, 1 out]
        }
        n175 = Bundle By Name(cluster=w457, "VISA name"=w454) -> (w456:T4)
      }
      frame "Wait" {
        n176 = Unbundle By Name(w480) -> ("VISA name"=w478:refnum<visa-resource-name>)
        n177 = Wait (ms)(milliseconds to wait=u32 50) -> ()  [unwired: 1 out]
        n178 = call "VISA Command.vi"("error in"=w481, "Command"="/1Q" ("String To Write"), "VISA name in"=w478) -> ("error out"=w468:errorcluster, "Return"=w474:string, "VISA name out"=w477:refnum<visa-resource-name>)  [unwired: 6 in]
        n179 = Match Pattern(string=w474, regular expression="/0") -> (after substring=w472:string)  [unwired: 1 in, 3 out]
        n180 = Bundle By Name(cluster=w480, "VISA name"=w477) -> (w479:T4)
        n181 = String Subset(string=w472, length (rest)=1 ("length (rest)")) -> (substring=w470:string)  [unwired: 1 in]
        n182 = Equal?(x=w470, y="`" ("x")) -> (x = y?=w467:bool)
        n183 = case shown="True" w467 {
          tunnel: w468 -> [w484 w486]
          tunnel: [w483 w486] -> w466
          tunnel: w465 -> [w485 _]
          frame False {
            n184 = call "Enqueue Prior.vi"("Error In"=w484, "State"="Wait", "Queue in"=w485) -> ("Error Out"=w483:errorcluster)  [unwired: 7 in, 1 out]
          }
          frame True {
          }
        }
      }
      frame "1stSetting" {
        n185 = Unbundle By Name(w491) -> ("VISA name"=w489:refnum<visa-resource-name>)
        n186 = call "VISA Command.vi"("error in"=w493, "Command"="/1aM4V500R" ("String To Write"), "VISA name in"=w489) -> ("error out"=w492:errorcluster, "VISA name out"=w488:refnum<visa-resource-name>)  [unwired: 6 in, 1 out]
        n187 = Bundle By Name(cluster=w491, "VISA name"=w488) -> (w490:T4)
      }
      frame "1stHome" {
        n188 = Unbundle By Name(w498) -> ("VISA name"=w496:refnum<visa-resource-name>)
        n189 = call "VISA Command.vi"("error in"=w500, "Command"="/1aM1P1000000aM2P1000000aM3P50000aM4P100000R" ("String To Write"), "VISA name in"=w496) -> ("error out"=w499:errorcluster, "VISA name out"=w495:refnum<visa-resource-name>)  [unwired: 6 in, 1 out]
        n190 = Bundle By Name(cluster=w498, "VISA name"=w495) -> (w497:T4)
      }
      frame "1stOutOfHome" {
        n191 = Unbundle By Name(w505) -> ("VISA name"=w503:refnum<visa-resource-name>)
        n192 = call "VISA Command.vi"("error in"=w507, "Command"="/1aM1D2000aM2D2000aM3D2000aM4D64R" ("String To Write"), "VISA name in"=w503) -> ("error out"=w506:errorcluster, "VISA name out"=w502:refnum<visa-resource-name>)  [unwired: 6 in, 1 out]
        n193 = Bundle By Name(cluster=w505, "VISA name"=w502) -> (w504:T4)
      }
      frame "2ndSetting" {
        n194 = Unbundle By Name(w512) -> ("VISA name"=w510:refnum<visa-resource-name>)
        n195 = call "VISA Command.vi"("error in"=w514, "Command"="/1aM1V10000aM2V10000aM3V10000aM4V10L10R" ("String To Write"), "VISA name in"=w510) -> ("error out"=w513:errorcluster, "VISA name out"=w509:refnum<visa-resource-name>)  [unwired: 6 in, 1 out]
        n196 = Bundle By Name(cluster=w512, "VISA name"=w509) -> (w511:T4)
      }
      frame "2ndHome" {
        n197 = Unbundle By Name(w519) -> ("VISA name"=w517:refnum<visa-resource-name>)
        n198 = call "VISA Command.vi"("error in"=w521, "Command"="/1aM1P1000000aM2P1000000aM3P50000aM4P100000R" ("String To Write"), "VISA name in"=w517) -> ("error out"=w520:errorcluster, "VISA name out"=w516:refnum<visa-resource-name>)  [unwired: 6 in, 1 out]
        n199 = Bundle By Name(cluster=w519, "VISA name"=w516) -> (w518:T4)
      }
      frame "2ndOutOfHome" {
        n200 = Unbundle By Name(w526) -> ("VISA name"=w524:refnum<visa-resource-name>)
        n201 = call "VISA Command.vi"("error in"=w528, "Command"="/1aM1D500aM2D500aM3D500aM4D100R" ("String To Write"), "VISA name in"=w524) -> ("error out"=w527:errorcluster, "VISA name out"=w523:refnum<visa-resource-name>)  [unwired: 6 in, 1 out]
        n202 = Bundle By Name(cluster=w526, "VISA name"=w523) -> (w525:T4)
      }
      frame "SetTo0" {
        n203 = Unbundle By Name(w533) -> ("VISA name"=w531:refnum<visa-resource-name>)
        n204 = call "VISA Command.vi"("error in"=w535, "Command"="/1z0,0,0,-200R" ("String To Write"), "VISA name in"=w531) -> ("error out"=w534:errorcluster, "VISA name out"=w530:refnum<visa-resource-name>)  [unwired: 6 in, 1 out]
        n205 = Bundle By Name(cluster=w533, "VISA name"=w530) -> (w532:T4)
      }
      frame "Position" {
        n206 = Unbundle By Name(w549) -> ("VISA name"=w547:refnum<visa-resource-name>)
        n207 = call "VISA Command.vi"("error in"=w550, "Command"="/1?aA", "VISA name in"=w547) -> ("error out"=w540:errorcluster, "Return"=w539:string, "VISA name out"=w546:refnum<visa-resource-name>)  [unwired: 6 in]
        n208 = Bundle By Name(cluster=w549, "VISA name"=w546) -> (w548:T4)
        n209 = call "Read String Convert.vi"("error in"=w540, "read string in"=w539) -> ("error out"=w538:errorcluster, "4position"=w536:i32[])  [unwired: 7 in, 1 out]
        "Current Position" <- w536
        n210 = call "SEQ Preview Queue.vi"("error in"=w538) -> ("error out"=w544:errorcluster, "SEQ Data"=w542:T9)  [unwired: 9 in]
        n211 = Bundle By Name(cluster=w542, "Position"=w536, "Arrived?"=TRUE) -> (w541:T9)
        n212 = call "SEQ Lossy Queue.vi"("error in"=w544, "SEQ Data"=w541) -> ("error out"=w543:errorcluster)  [unwired: 9 in]
      }
      frame "Move" {
        n213 = Unbundle By Name(w559) -> ("VISA name"=w557:refnum<visa-resource-name>)
        n214 = Variant To Data(error in=w555, type="", Variant=w553) -> (data=w551:string, error out=w554:errorcluster)
        n215 = call "VISA Command.vi"("error in"=w554, "Command"=w551, "VISA name in"=w557) -> ("error out"=w560:errorcluster, "VISA name out"=w556:refnum<visa-resource-name>)  [unwired: 6 in, 1 out]
        n216 = Bundle By Name(cluster=w559, "VISA name"=w556) -> (w558:T4)
      }
      frame "Joystick" {
        n217 = Unbundle By Name(w569) -> ("VISA name"=w567:refnum<visa-resource-name>)
        n218 = Variant To Data(error in=w565, type="", Variant=w563) -> (data=w561:string, error out=w564:errorcluster)
        n219 = call "VISA Command.vi"("error in"=w564, "Command"=w561, "VISA name in"=w567) -> ("error out"=w570:errorcluster, "VISA name out"=w566:refnum<visa-resource-name>)  [unwired: 6 in, 1 out]
        n220 = Bundle By Name(cluster=w569, "VISA name"=w566) -> (w568:T4)
      }
      frame "Delay" {
        n221 = Variant To Data(error in=w575, type=u32 0 ("milliseconds to wait"), Variant=w574) -> (data=w571:u32, error out=w573:errorcluster)
        n222 = Wait (ms)(milliseconds to wait=w571) -> ()  [unwired: 1 out]
      }
      frame "Emergency Stop" {
        n223 = Unbundle By Name(w583) -> ("VISA name"=w581:refnum<visa-resource-name>)
        n224 = Wait (ms)(milliseconds to wait=u32 200) -> ()  [unwired: 1 out]
        n225 = call "VISA Command.vi"("error in"=w579, "Command"="/1T", "VISA name in"=w581) -> ("error out"=w584:errorcluster, "VISA name out"=w580:refnum<visa-resource-name>)  [unwired: 6 in, 1 out]
        n226 = Bundle By Name(cluster=w583, "VISA name"=w580) -> (w582:T4)
      }
      frame "Rendezvous Acquire" {
        n227 = call <vilib>:"Create Rendezvous.vi"("error in (no error)"=w593, "size (2)"=4, "name (unnamed)"="Acquire") -> ("error out"=w592:errorcluster, "rendezvous"=w589:T10)  [unwired: 2 in, 1 out]
        n228 = call <vilib>:"Wait at Rendezvous.vi"("error in (no error)"=w592, "ms timeout (-1)"=10000, "rendezvous"=w589) -> ("error out"=w587:errorcluster, "timed out"=w586:bool)  [unwired: 2 in, 1 out]
        n229 = case shown="True" w586 {
          tunnel: w587 -> [w595 _]
          tunnel: [w595 w596] -> w585
          frame False {
          }
          frame True {
            n230 = xnode "Error Ring"() -> ("error out"=w596:errorcluster)
          }
        }
      }
      frame "Rendezvous Focus" {
        n231 = call <vilib>:"Create Rendezvous.vi"("error in (no error)"=w610, "size (2)"=2, "name (unnamed)"="Focus") -> ("error out"=w609:errorcluster, "rendezvous"=w606:T10)  [unwired: 2 in, 1 out]
        n232 = call <vilib>:"Wait at Rendezvous.vi"("error in (no error)"=w609, "ms timeout (-1)"=10000, "rendezvous"=w606) -> ("error out"=w604:errorcluster, "timed out"=w603:bool)  [unwired: 2 in, 1 out]
        n233 = case shown="True" w603 {
          tunnel: w604 -> [w612 _]
          tunnel: [w612 w613] -> w602
          frame False {
          }
          frame True {
            n234 = xnode "Error Ring"() -> ("error out"=w613:errorcluster)
          }
        }
      }
      frame "Rendezvous Align" {
        n235 = call <vilib>:"Create Rendezvous.vi"("error in (no error)"=w627, "size (2)"=2, "name (unnamed)"="Align") -> ("error out"=w626:errorcluster, "rendezvous"=w623:T10)  [unwired: 2 in, 1 out]
        n236 = call <vilib>:"Wait at Rendezvous.vi"("error in (no error)"=w626, "ms timeout (-1)"=10000, "rendezvous"=w623) -> ("error out"=w621:errorcluster, "timed out"=w620:bool)  [unwired: 2 in, 1 out]
        n237 = case shown="True" w620 {
          tunnel: w621 -> [w629 _]
          tunnel: [w629 w630] -> w619
          frame False {
          }
          frame True {
            n238 = xnode "Error Ring"() -> ("error out"=w630:errorcluster)
          }
        }
      }
      frame "Rotate U" {
        n239 = Unbundle By Name(w651) -> ("VISA name"=w649:refnum<visa-resource-name>, "Dichroic Position"=w643:string[])
        n240 = Variant To Data(error in=w647, type=enum16{"1", "2", "3", "4", "5", "6", "7", "8"}."1" ("Cube"), Variant=w645) -> (data=w638:enum16{"1", "2", "3", "4", "5", "6", "7", "8"}, error out=w646:errorcluster)
        n241 = To Unsigned Word Integer(number=w638) -> (unsigned 16bit integer=w637:u16)
        n242 = Index Array(array=w643, index=w637) -> (element=w640:string)
        n243 = case shown="0, Default" w637 {
          tunnel: [T1."Cube 1" ("Cube") T1."Cube 2" ("Cube") T1."Cube 3" ("Cube") T1."Cube 4" ("Cube") T1."Cube 5" ("Cube") T1."Cube 6" ("Cube") T1."Cube 7" ("Cube") T1."Cube 8" ("Cube")] -> w636
          frame 0, Default {
          }
          frame 1 {
          }
          frame 2 {
          }
          frame 3 {
          }
          frame 4 {
          }
          frame 5 {
          }
          frame 6 {
          }
          frame 7 {
          }
        }
        n244 = Concatenate Strings("/1aM4A", w640, "R" ("string")) -> (w639:string)
        n245 = property on="Cube" class="RadioBtnsControl (strict)"("Value"=w636) -> ()  [unwired: 2 in, 2 out]
        n246 = call "VISA Command.vi"("error in"=w646, "Command"=w639, "VISA name in"=w649) -> ("error out"=w652:errorcluster, "VISA name out"=w648:refnum<visa-resource-name>)  [unwired: 6 in, 1 out]
        n247 = Bundle By Name(cluster=w651, "VISA name"=w648) -> (w650:T4)
      }
      frame "Position Continue" {
        n248 = Unbundle By Name(w678) -> ("VISA name"=w676:refnum<visa-resource-name>)
        n249 = call "Enqueue.vi"("Error In"=w665, "State"="Position Continue", "Queue in"=w663) -> ("Error Out"=w664:errorcluster)  [unwired: 7 in, 1 out]
        n250 = Wait (ms)(milliseconds to wait=u32 200) -> ()  [unwired: 1 out]
        n251 = call "VISA Command.vi"("error in"=w664, "Command"="/1?aA", "VISA name in"=w676) -> ("error out"=w669:errorcluster, "Return"=w668:string, "VISA name out"=w675:refnum<visa-resource-name>)  [unwired: 6 in]
        n252 = Bundle By Name(cluster=w678, "VISA name"=w675) -> (w677:T4)
        n253 = call "Read String Convert.vi"("error in"=w669, "read string in"=w668) -> ("error out"=w667:errorcluster, "4position"=w666:i32[])  [unwired: 7 in, 1 out]
        n254 = local write "Current Position"(w666) -> ()
        n255 = call "SEQ Preview Queue.vi"("error in"=w667) -> ("error out"=w673:errorcluster, "SEQ Data"=w671:T9)  [unwired: 9 in]
        n256 = Bundle By Name(cluster=w671, "Position"=w666) -> (w670:T9)
        n257 = call "SEQ Lossy Queue.vi"("error in"=w673, "SEQ Data"=w670) -> ("error out"=w672:errorcluster)  [unwired: 9 in]
      }
      frame "Go Reference" {
        n258 = Unbundle By Name(w690) -> ("VISA name"=w688:refnum<visa-resource-name>, "Reference"=w685:string[])
        n259 = Index Array(array=w685) -> (element #1=w681:string, element #2=w680:string)  [unwired: 2 in]
        n260 = Concatenate Strings("/1aM1A", w681, "aM2A", w680, "R") -> (w679:string)
        n261 = call "VISA Command.vi"("error in"=w686, "Command"=w679, "VISA name in"=w688) -> ("error out"=w691:errorcluster, "VISA name out"=w687:refnum<visa-resource-name>)  [unwired: 6 in, 1 out]
        n262 = Bundle By Name(cluster=w690, "VISA name"=w687) -> (w689:T4)
      }
      frame "------Error Handler------" {
      }
      frame "Error" {
        n263 = Variant To Data(error in=w698, type=errorcluster {"status"=FALSE, "code"=0, "source"=""} ("error constant"), Variant=w697) -> (data=w695:errorcluster)  [unwired: 1 out]
        n264 = call <vilib>:"Simple Error Handler.vi"("error in (no error)"=w695) -> ()  [unwired: 4 in, 5 out]
      }
      frame "------Close------" {
      }
      frame "Close" {
        n265 = for {
          tunnel: w704 -> [w708]
          shift-right: [w709] -> w705
          shift-left: w706 -> [w710]
          tunnel: string[] ["Close Device", "Release Queue"] -> [w707] mode=indexing
          n266 = call "Enqueue.vi"("Error In"=w710, "State"=w707, "Queue in"=w708) -> ("Error Out"=w709:errorcluster)  [unwired: 7 in, 1 out]
        }
      }
      frame "Close Device" {
        n267 = Unbundle By Name(w712) -> ("VISA name"=w711:refnum<visa-resource-name>)
        n268 = VISA Close(VISA resource name=w711, error in (no error)=w714) -> (error out=w713:errorcluster)
      }
      frame "Release Queue" {
        n269 = Release Queue(queue=w719, error in (no error)=w720) -> (error out=w716:errorcluster)  [unwired: 1 in, 2 out]
        n270 = call "SEQ Release Queue.vi"("error in"=w716) -> ("error out"=w715:errorcluster)  [unwired: 10 in]
      }
    }
    n271 = case shown="Error .." w341 {
      selector: w341 -> [w345 w349]
      tunnel: [w345 w350] -> w340
      tunnel: w339 -> [_ w347]
      frame No Error {
      }
      frame Error {
        n272 = To Variant(anything=w349) -> (Variant=w348:variant)
        n273 = call "Enqueue.vi"("Data"=w348, "State"="Error", "Queue in"=w347) -> ("Error Out"=w350:errorcluster)  [unwired: 7 in, 1 out]
      }
    }
  }
  n274 = Merge Errors(w10, w8) -> (→"error out":errorcluster)
